vi "kinectOpen.vi"() -> (0 "error out":errorcluster, 3 "KinectSensor References":T1)   [LabVIEW 2014]
uses:
  Controls/KinectSensor References.ctl
  Microsoft.Kinect
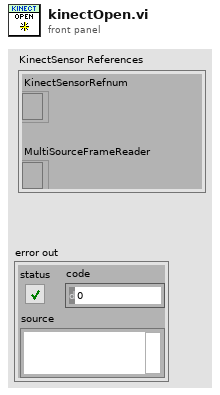
[diagram p1: front panel]
types:
  T1 = typedef "KinectSensor References.ctl" = cluster{"KinectSensorRefnum":refnum<k24>, "MultiSourceFrameReader":refnum<k24>}
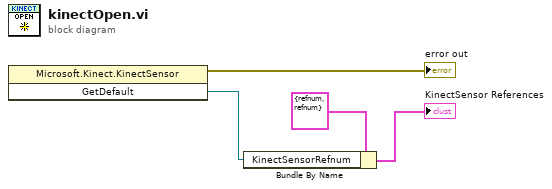
[diagram p0: block diagram]
diagram:
  n1 = invoke on="Invoke Node" class="Microsoft.Kinect.KinectSensor" method="GetDefault"() -> (error out=→"error out":errorcluster, "GetDefault"=w3:refnum<k24>)  [unwired: 3 in, 1 out]
  n2 = Bundle By Name(cluster=T1 {"KinectSensorRefnum"=refnum, "MultiSourceFrameReader"=refnum} ("KinectSensor References"), "KinectSensorRefnum"=w3) -> (→"KinectSensor References":T1)
